vi "update exposure time slider.vi"(8 "error in (no error)":errorcluster, 11 "Thorcam in":refnum<class "Thorcam.lvclass">) -> (0 "error out":errorcluster, 3 "Thorcam out":refnum<class "Thorcam.lvclass">)   [LabVIEW 2012, in "Thorcam.lvclass"]
uses:
  Thorcam.lvclass
  Thorcam.lvclass/Thorcam.ctl
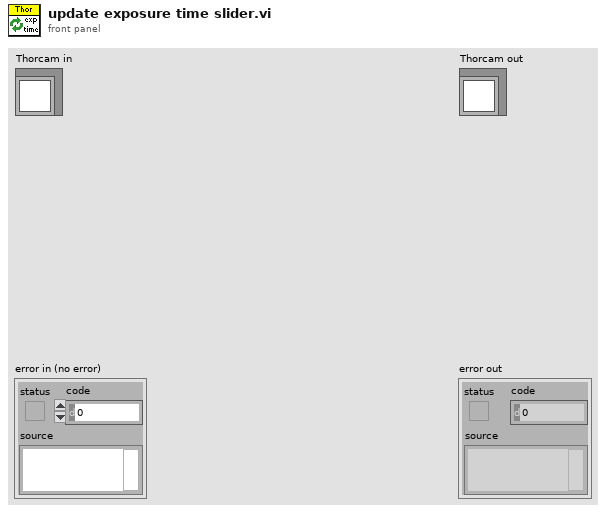
[diagram p1: front panel]
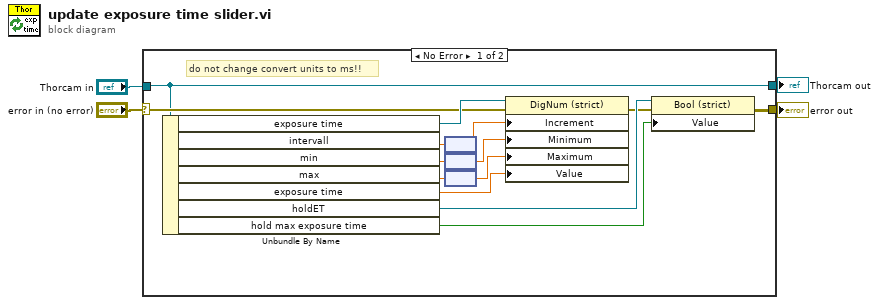
[diagram p0: block diagram]
diagram:
  n1 = case shown="No Error" "error in (no error)" {
    selector: "error in (no error)" -> [w11 w20]
    tunnel: [w6 w20] -> w3
    tunnel: [w10 w19] -> w1
    tunnel: "Thorcam in" -> [w10 w19]
    frame No Error {
      # "do not change convert units to ms!!"
      n2 = Unbundle By Name(w10) -> ("exposure time"=w18:refnum<vi>, "intervall"=w17:dbl[unit], "min"=w16:dbl[unit], "max"=w15:dbl[unit], "exposure time"=w9:dbl[unit], "holdET"=w8:refnum<vi>, "hold max exposure time"=w5:bool)
      n3 = node(w17) -> (w12:dbl)
      n4 = node(w16) -> (w14:dbl)
      n5 = node(w15) -> (w13:dbl)
      n6 = property class="DigNum (strict)"(reference=w18, error in=w11, "Increment"=w12, "Minimum"=w14, "Maximum"=w13, "Value"=w9) -> (error out=w7:errorcluster)  [unwired: 1 out]
      n7 = property class="Bool (strict)"(reference=w8, error in=w7, "Value"=w5) -> (error out=w6:errorcluster)  [unwired: 1 out]
    }
    frame Error {
    }
  }
  "error out" <- w3
  "Thorcam out" <- w1
